vi "User and Password.vi"(8 "error in (no error)":errorcluster, 11 "Path":path=path "C:/Users/15889/Desktop/TP3_FTT/system") -> (0 "error out":errorcluster, 3 "output cluster":T1)   [LabVIEW 2014]
panel:
  in  "Quit":bool
  in  "OK":bool
  in  "Password":string caption="密    码："
  in  "UserName":string caption="用户名："
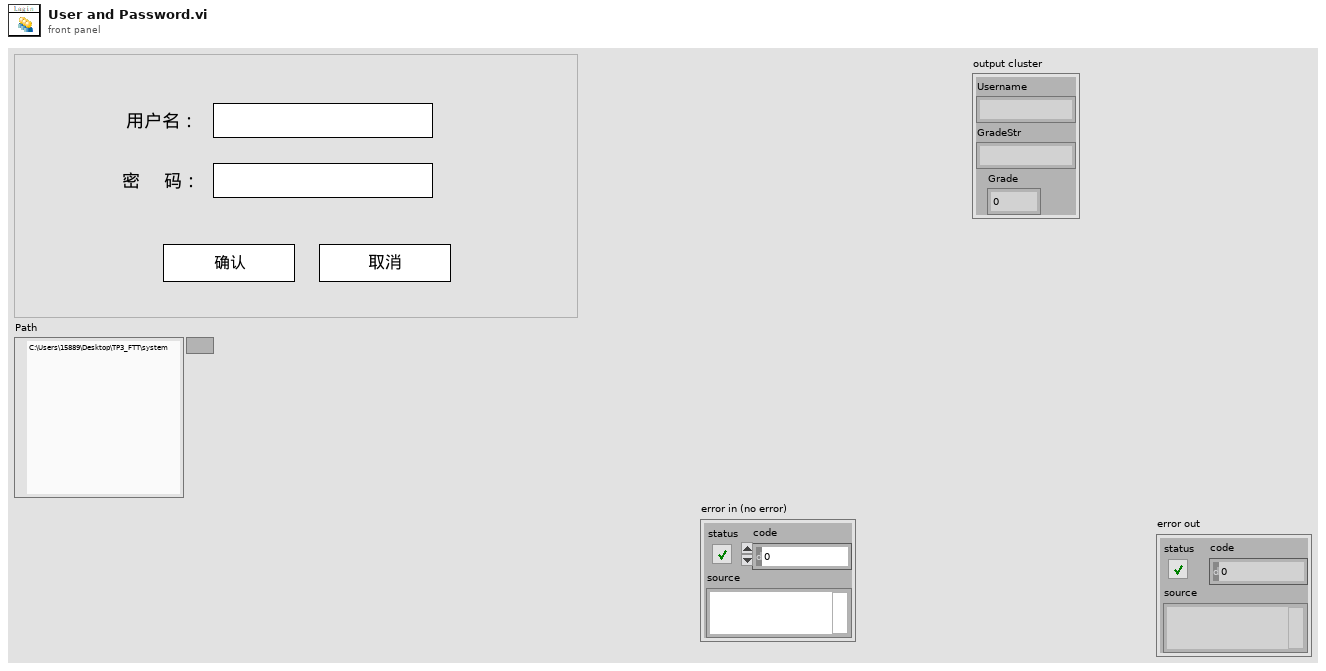
[diagram p1: front panel]
types:
  T1 = cluster{"Username":string, "GradeStr":string, "Grade":u32}
  T2 = cluster{"Username":string, "Password":string, "Grade":u32}
  T3 = cluster{"Username":string, "Password":string, "Grade":u32}[]
  T4 = cluster{"Login":cluster{"Username":string, "Password":string, "Grade":u32}, "U&P":cluster{"Username":string, "Password":string, "Grade":u32}[], "Quit":refnum<vi>, "OK":refnum<vi>, "Password":refnum<vi>, "UserName":refnum<vi>, "Path":path}
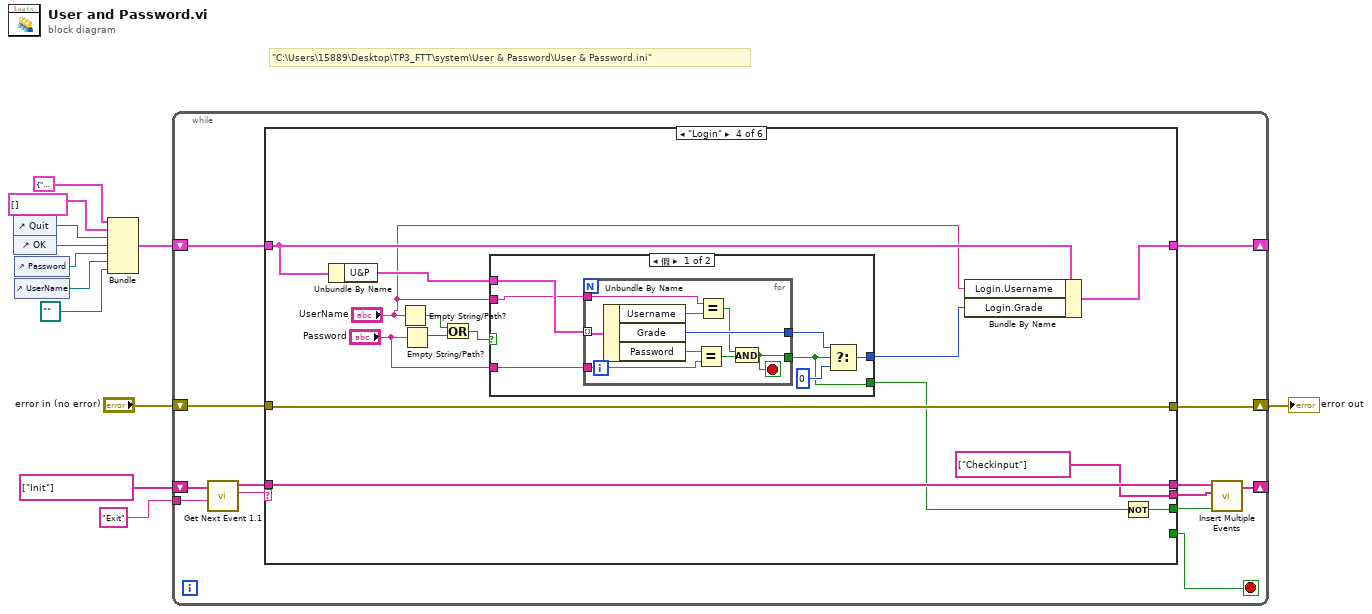
[diagram p0: block diagram]
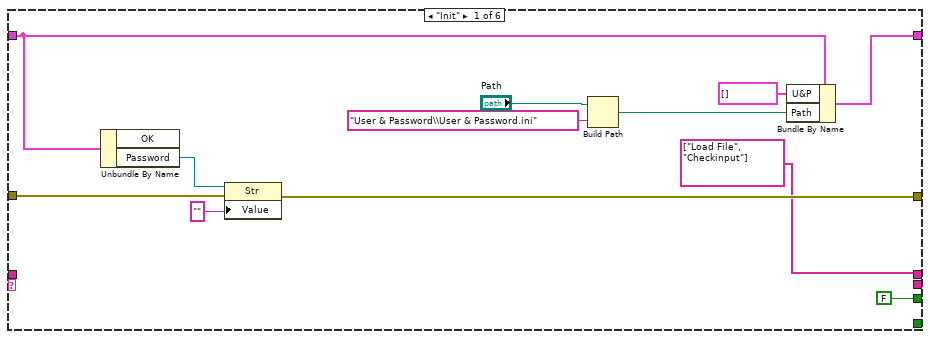
[diagram p2: hidden frame]
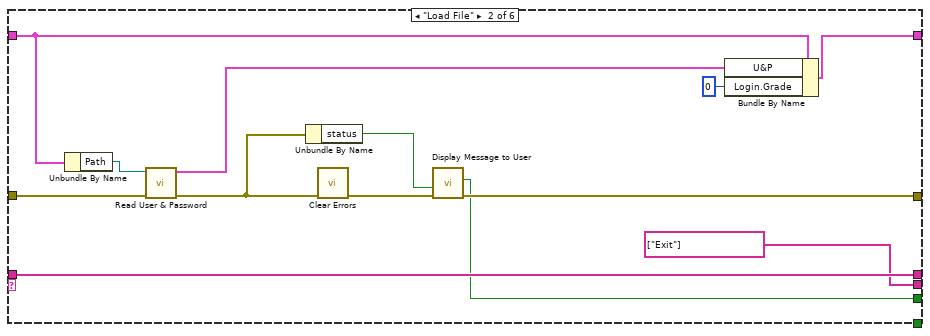
[diagram p3: hidden frame]
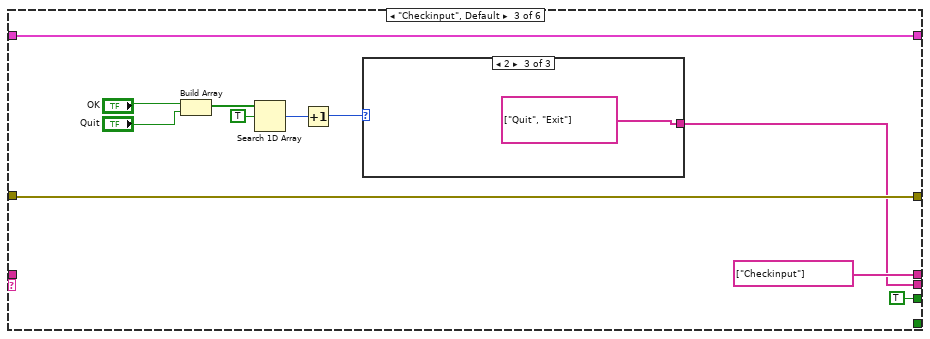
[diagram p4: hidden frame]
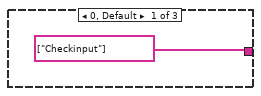
[diagram p5: hidden frame]
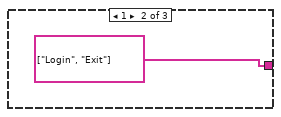
[diagram p6: hidden frame]
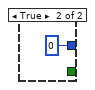
[diagram p7: hidden frame]
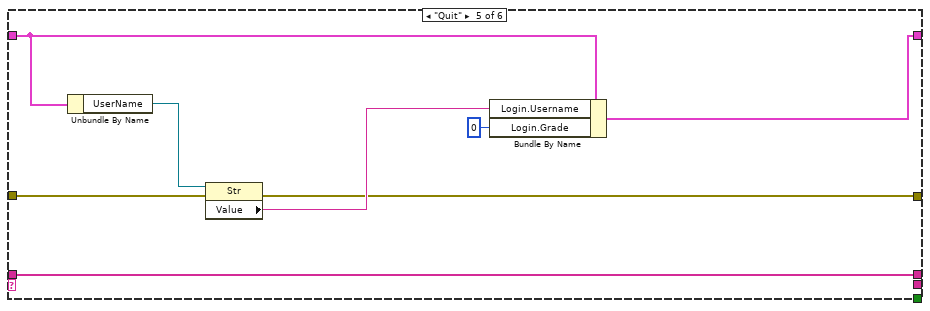
[diagram p8: hidden frame]
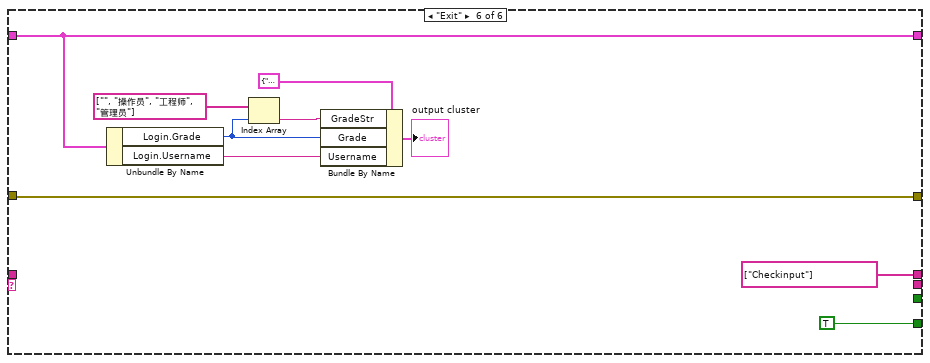
[diagram p9: hidden frame]
diagram:
  # "\"C:\\Users\\15889\\Desktop\\TP3_FTT\\system\\User & Password\\User & Password.ini\""
  n1 = control-ref of="Quit"() -> (w10:refnum<vi>)
  n2 = control-ref of="OK"() -> (w9:refnum<vi>)
  n3 = control-ref of="Password"() -> (w8:refnum<vi>)
  n4 = control-ref of="UserName"() -> (w7:refnum<vi>)
  n5 = Bundle("Login"=T2 {"Username"="", "Password"="", "Grade"=0}, "U&P"=T3 [], "Quit"=w10, "OK"=w9, "Password"=w8, "UserName"=w7, "Path"=path "") -> (w5:T4)  [unwired: 1 in]
  n6 = while {
    shift-right: [w21] -> _
    shift-left: string[] ["Init"] -> [w24]
    tunnel: "Exit" -> [w22]
    shift-right: [w18] -> _
    shift-left: w5 -> [w19]
    shift-right: [w16] -> w3
    shift-left: "error in (no error)" -> [w17]
    stop <- w13 stop-if-true
    n7 = call "Get Next Event 1.1.vi"("Exit Event"=w22, "event queue in"=w24) -> ("next event"=w25:string, "event queue out"=w23:string[])  [unwired: 6 in, 2 out]
    n8 = case shown="\"Login\"" w25 {
      tunnel: w23 -> [_ w50 _ w68 w102 _]
      tunnel: [string[] ["Load File", "Checkinput"] w50 string[] ["Checkinput"] w68 w102 string[] ["Checkinput"]] -> w20
      tunnel: w19 -> [w35 w47 w61 w72 w101 w110]
      tunnel: [w36 w45 w61 w71 w103 w110] -> w18
      tunnel: w17 -> [w34 w49 w60 w76 w100 w113]
      tunnel: [w30 w42 w60 w76 w97 w113] -> w16
      tunnel: [FALSE w41 TRUE ("OK") w67 _ _] -> w15
      tunnel: [_ string[] ["Exit"] w52 string[] ["Checkinput"] _ _] -> w14
      tunnel: [_ _ _ _ _ TRUE] -> w13
      frame "Init" {
        n9 = Unbundle By Name(w35) -> ("Password"=w33:refnum<vi>)  [unwired: 1 out]
        n10 = property class="Str"(reference=w33, error in=w34, "Value"="") -> (error out=w30:errorcluster)  [unwired: 1 out]
        n11 = Build Path(base path="Path", name or relative path="User & Password\\User & Password.ini") -> (appended path=w28:path)
        n12 = Bundle By Name(cluster=w35, "U&P"=T3 [], "Path"=w28) -> (w36:T4)
      }
      frame "Load File" {
        n13 = Unbundle By Name(w47) -> ("Path"=w48:path)
        n14 = call "Read User & Password.vi"("error in (no error)"=w49, "Path"=w48) -> ("error out"=w40:errorcluster, "Array"=w46:cluster{"value":string, "value":string, i32}[])  [unwired: 8 in]
        n15 = Unbundle By Name(w40) -> ("status"=w43:bool)
        n16 = call <vilib>:"Clear Errors.vi"("error in (no error)"=w40) -> ("error out"=w39:errorcluster)  [unwired: 5 in, 1 out]
        n17 = call "Display Message to User"("error in (no error)"=w39, "Enable"=w43) -> ("error out"=w42:errorcluster, "OK"=w41:bool)  [unwired: 8 in]
        n18 = Bundle By Name(cluster=w47, "U&P"=w46, "Login.Grade"=u32 0) -> (w45:T4)
      }
      frame "Checkinput", Default {
        n19 = Build Array("OK", "Quit") -> (w57:bool[])
        n20 = Search 1D Array(1D array=w57, element=TRUE) -> (index of element=w54:i32)  [unwired: 1 in]
        n21 = Increment(x=w54) -> (x+1=w53:i32)
        n22 = case shown="2" w53 {
          tunnel: [string[] ["Checkinput"] string[] ["Login", "Exit"] string[] ["Quit", "Exit"]] -> w52
          frame 0, Default {
          }
          frame 1 {
          }
          frame 2 {
          }
        }
      }
      frame "Login" {
        n23 = Unbundle By Name(w72) -> ("U&P"=w73:T3)
        n24 = Empty String/Path?(string/path="UserName") -> (empty?=w77:bool)
        n25 = Empty String/Path?(string/path="Password") -> (empty?=w78:bool)
        n26 = Or(x=w77, y=w78) -> (x .or. y?=w75:bool)
        n27 = case shown="假" w75 {
          tunnel: "UserName" -> [w84 _]
          tunnel: "Password" -> [w83 _]
          tunnel: w73 -> [w85 _]
          tunnel: [w80 u32 0 ("f")] -> w70
          tunnel: [w79 _] -> w66
          frame False {
            n28 = for {
              tunnel: w85 -> [w94] mode=indexing
              tunnel: w84 -> [w92]
              tunnel: w83 -> [w90]
              tunnel: [w89] -> w82
              tunnel: [w86] -> w79
              stop <- w86 stop-if-true
              n29 = Unbundle By Name(w94) -> ("Username"=w93:string, "Grade"=w89:u32, "Password"=w91:string)
              n30 = Equal?(x=w91, y=w90) -> (x = y?=w88:bool)
              n31 = Equal?(x=w92, y=w93) -> (x = y?=w87:bool)
              n32 = And(x=w87, y=w88) -> (x .and. y?=w86:bool)
            }
            n33 = Select(t=w82, s=w79, f=u32 0) -> (s? t:f=w80:u32)
          }
          frame True {
          }
        }
        n34 = Bundle By Name(cluster=w72, "Login.Username"="UserName", "Login.Grade"=w70) -> (w71:T4)
        n35 = Not(x=w66) -> (.not. x?=w67:bool)
      }
      frame "Quit" {
        n36 = Unbundle By Name(w101) -> ("UserName"=w99:refnum<vi>)
        n37 = property class="Str"(reference=w99, error in=w100) -> (error out=w97:errorcluster, "Value"=w98:string)  [unwired: 1 out]
        n38 = Bundle By Name(cluster=w101, "Login.Username"=w98, "Login.Grade"=u32 0) -> (w103:T4)
      }
      frame "Exit" {
        n39 = Unbundle By Name(w110) -> ("Login.Grade"=w106:u32, "Login.Username"=w105:string)
        n40 = Index Array(array=string[] ["", "操作员", "工程师", "管理员"], index=w106) -> (element=w107:string)
        n41 = Bundle By Name(cluster=T1 {"Username"="", "GradeStr"="", "Grade"=0} ("Login"), "GradeStr"=w107, "Grade"=w106, "Username"=w105) -> (→"output cluster":T1)
      }
    }
    n42 = call "Insert Multiple Events.vi"("Insert all? (T)"=w15, "Events to Insert"=w14, "Event queue in"=w20) -> ("Event queue out"=w21:string[])  [unwired: 4 in]
  }
  "error out" <- w3
